vi "Get Header.vi"(8 "error in":errorcluster, 10 "header":T1, 11 "session in":refnum<class "Session.lvclass">) -> (0 "error out":errorcluster, 2 "value":string, 3 "session out":refnum<class "Session.lvclass">)   [LabVIEW 2019, in "NI_Advanced HTTP Client.lvlib" / "Session.lvclass"]
doc: "Returns the value assigned to the header of the HTTP session. Headers define attributes of the data exchanged between the client and server."
uses:
  Session.lvclass
  Header--Combo Box.ctl
  Session.lvclass/Session.ctl
  lvwebclient_64.dll
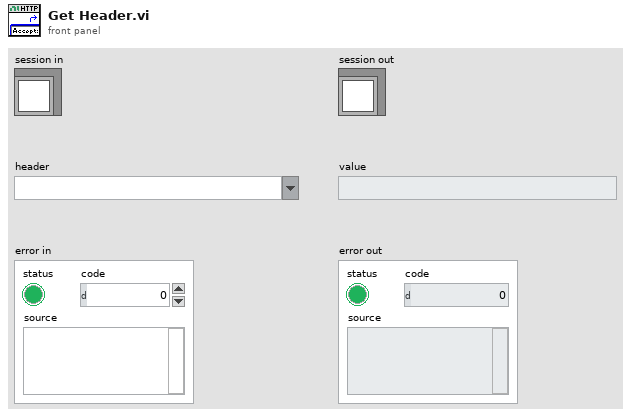
[diagram p1: front panel]
types:
  T1 = typedef "NI_Advanced HTTP Client.lvlib/Session.lvclass/Header--Combo Box.ctl" = string
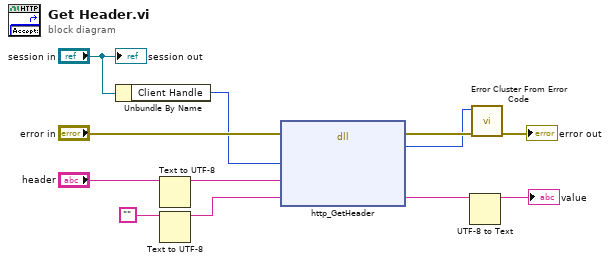
[diagram p0: block diagram]
diagram:
  n1 = Unbundle By Name("session in") -> ("Client Handle"=w6:u32)
  n2 = Text to UTF-8(11:"header") -> (3:w5:string)  [unwired: 2 in, 1 out]
  n3 = Text to UTF-8(11:"") -> (3:w3:string)  [unwired: 2 in, 1 out]
  n4 = dll-call lib="C:/Users/Localization Tester/Desktop/Advanced HTTP Client/lvwebclient_*.*" fn="http_GetHeader"(error in="error in", "handle"=w6, "headerName"=w5, "headerValue"=w3) -> (error out=w8:errorcluster, "return"=w7:i32, "headerValue"=w2:string)  [unwired: 4 in, 1 out]
  n5 = UTF-8 to Text(11:w2) -> (3:→"value":string)  [unwired: 2 in, 1 out]
  n6 = call <vilib>:"Error Cluster From Error Code.vi"("error in (no error)"=w8, "error code (0)"=w7) -> ("error out"=→"error out":errorcluster)  [unwired: 7 in]
  "session out" <- "session in"
